vi "Synth Program Outputs.vi"(2 "Match clocks":bool=TRUE, 4 "Use hardware clock for DO":bool, 5 "Mode":T2(ring), 6 "IF (Hz)":dbl=1000.0, 7 "Phase (degrees)":dbl min=0.0 max=360.0 step=11.25, 8 "error in (no error)":errorcluster, 9 "Clock Multiplier":i32=64, 10 "DAQmx Device Name":tag="6251", 11 "f (Hz)":dbl) -> (0 "error out":errorcluster, 3 "Actual ratios":T1 {"Clock" format="%_20p"; "F2" format="%_20p"; "F1" format="%_20p"; "Clock/F2" format="%_20g"; "Clock/F1" format="%_20g"})   [LabVIEW 2016]
uses:
  Actual Settings.ctl
  <vilib>/DAQmx/write.llb/DAQmx Write (Digital 1D U8 1Chan NSamp).vi
  <vilib>/DAQmx/miscellaneous.llb/DAQmx Fill In Error Info.vi
panel:
  out "Full Byte Array":u8[](array[numeric]) format="%08b"
  in  "Delay (ms)":u32=1
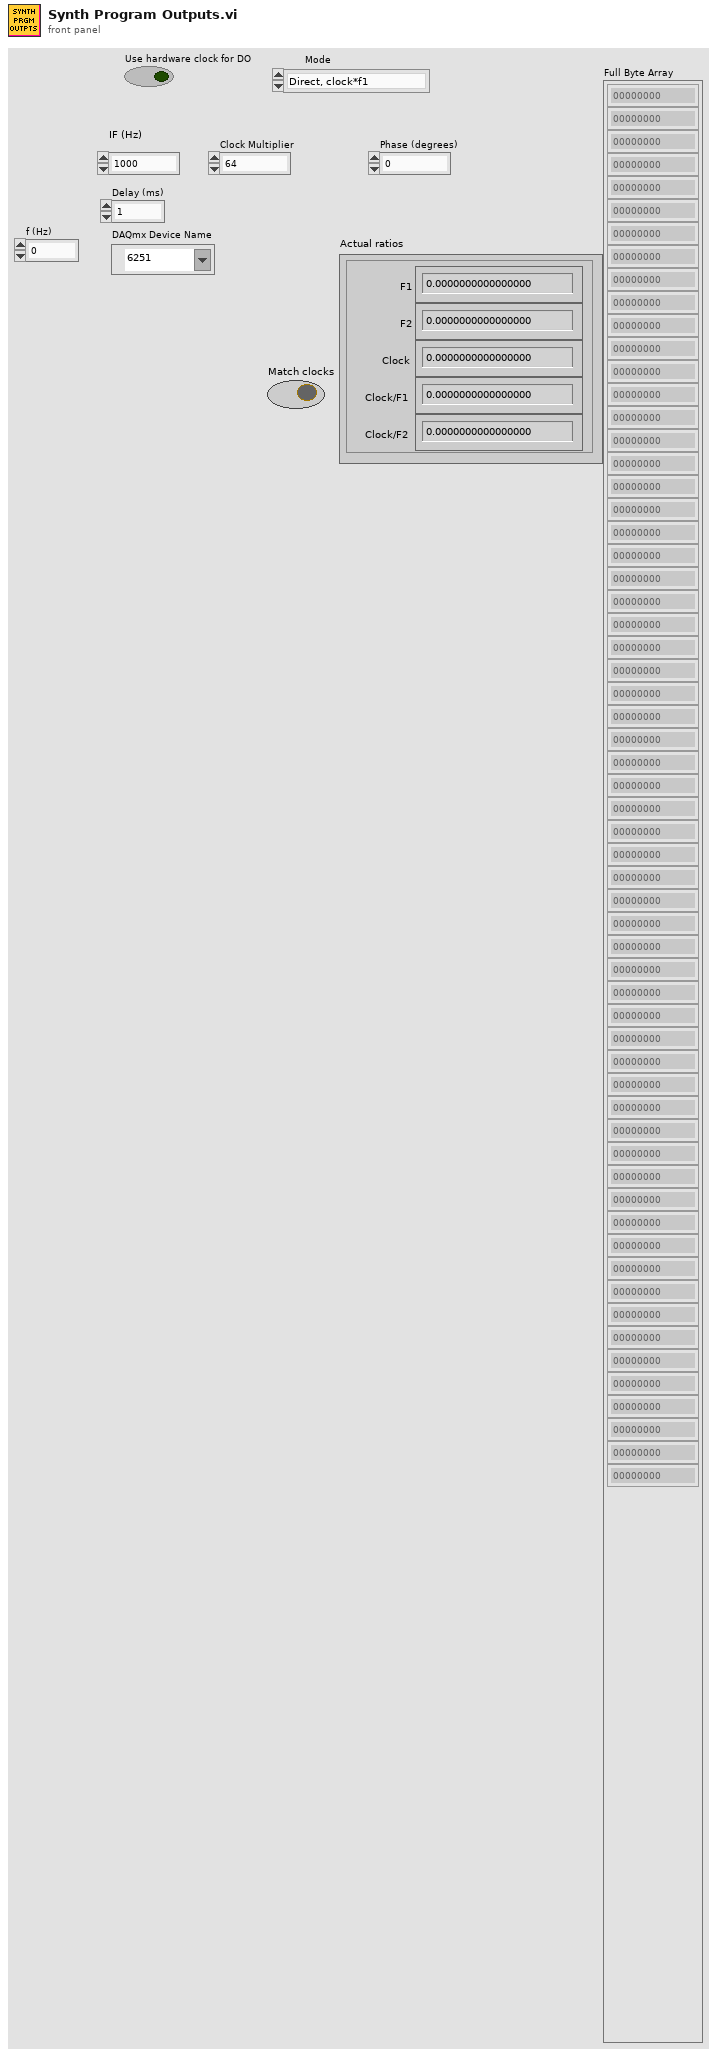
[diagram p1: front panel]
types:
  T1 = typedef "Actual settings.ctl" = cluster{"Clock/F1":ext, "Clock/F2":ext, "F1":ext, "F2":ext, "Clock":ext}
  T2 = enum16{"Direct, clock*f1", "Direct, clock*f2", "Heterodyne"}
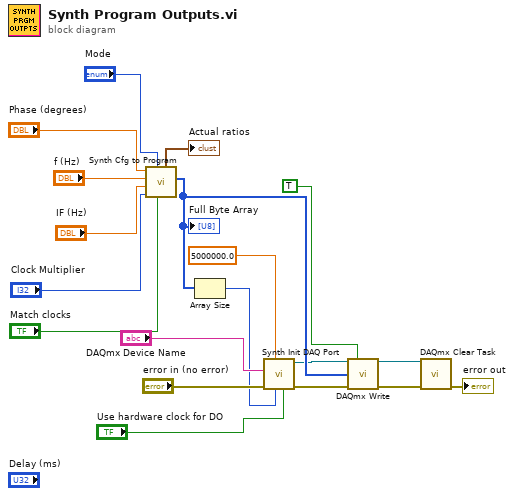
[diagram p0: block diagram]
diagram:
  n1 = call "Synth Cfg to Program.vi"("Match clocks"="Match clocks", "Mode"="Mode", "Clock Multiplier"="Clock Multiplier", "IF (Hz)"="IF (Hz)", "f (Hz)"="f (Hz)", "Phase (degrees)"="Phase (degrees)") -> ("Full Byte Array"=w8:u8[], "Actual ratios"=→"Actual ratios":T1)  [unwired: 2 in, 2 out]
  "Full Byte Array" <- w8
  n2 = Array Size(array=w8) -> (size(s)=w10:i32)
  n3 = call "Synth Init DAQ Port.vi"("Use hardware clock for DO"="Use hardware clock for DO", "DO Samples per Channel"=w10, "DO Clock Rate (Hz)"=5000000.0 ("Sample Clock Rate (Hz)"), "error in (no error)"="error in (no error)", "DAQmx Device Name"="DAQmx Device Name") -> ("error out"=w5:errorcluster, "task out"=w4:refnum<k21>)  [unwired: 5 in]
  n4 = call-poly <vilib>:"DAQmx Write.vi"("task/channels in"=w4, "auto start"=TRUE, "data"=w8, "error in"=w5) -> ("task out"=w6:refnum<k21>, "error out"=w7:errorcluster)  [unwired: 9 in, 1 out]
  n5 = call <vilib>:"DAQmx Clear Task.vi"("task in"=w6, "error in"=w7) -> ("error out"=→"error out":errorcluster)  [unwired: 13 out]
